vi "XNET Future Time Trigger.vi"(0 "session in":refnum<k21>, 5 "when":timestamp, 7 "timescale (local)":T1 items=["Local Time", "Network Time"], 11 "error in (no error)":errorcluster) -> (4 "session out":refnum<k21>, 15 "error out":errorcluster)   [LabVIEW 2018]
doc: "Provides the future timestamp for an exported Time Trigger."
uses:
  XNET Timescale.ctl
  nixlvapi.dll
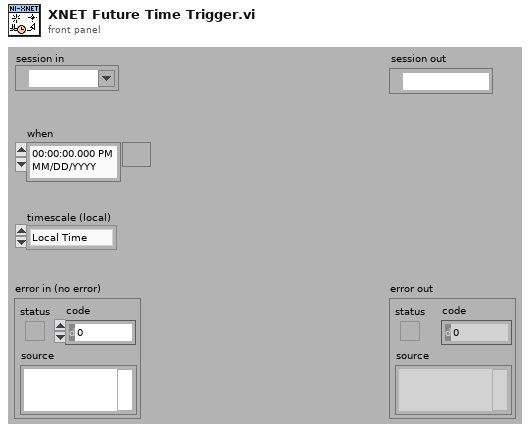
[diagram p1: front panel]
types:
  T1 = typedef "XNET Timescale.ctl" = u32
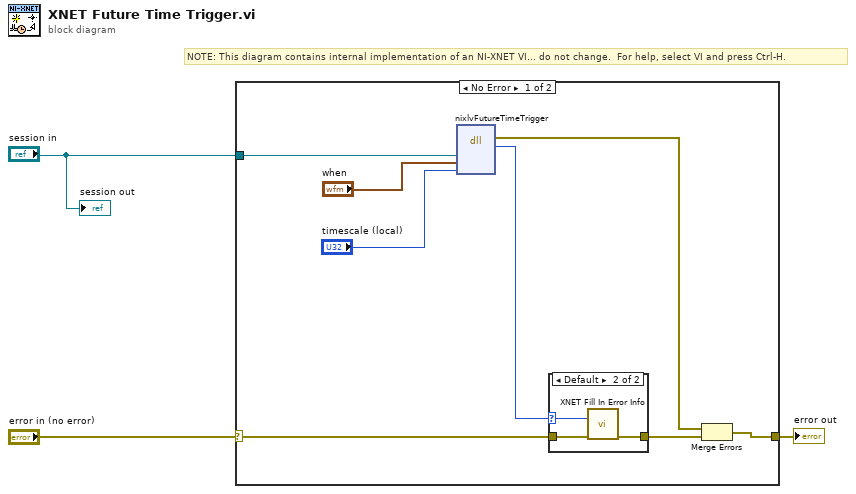
[diagram p0: block diagram]
diagram:
  # "NOTE: This diagram contains internal implementation of an NI-XNET VI... do not change.  For help, select VI and press Ctrl-H."
  n1 = case shown="No Error" "error in (no error)" {
    selector: "error in (no error)" -> [w10 w16]
    tunnel: "session in" -> [w11 _]
    tunnel: [w8 w16] -> w3
    frame No Error {
      n2 = dll-call lib="nixlvapi.*" fn="nixlvFutureTimeTrigger"("SessionRef"=w11, "when"="when", "timescale"="timescale (local)") -> (error out=w7:errorcluster, "return type"=w9:i32)  [unwired: 5 in, 2 out]
      n3 = case shown="Default" w9 {
        selector: w9 -> [_ w13]
        tunnel: w10 -> [w12 w14]
        tunnel: [w12 w15] -> w6
        frame 0 {
        }
        frame Default {
          n4 = call "XNET Fill In Error Info.vi"("status code"=w13, "error in"=w14) -> ("error out"=w15:errorcluster)  [unwired: 13 out]
        }
      }
      n5 = Merge Errors(w7, w6) -> (w8:errorcluster)
    }
    frame Error {
    }
  }
  "error out" <- w3
  "session out" <- "session in"
